vi "Launcher.vi"() -> ()   [LabVIEW 2019]
uses:
  <vilib>/ActorFramework/Message Enqueuer/Message Enqueuer.lvclass
  GUI Actor/GUI Actor.lvclass
  C:/Program Files (x86)/National Instruments/LabVIEW 2019/vi.lib/ActorFramework/Actor/Actor.lvclass
  ContadorB.lvclass
  <vilib>/ActorFramework/Message Enqueuer/Message Enqueuer.lvclass/Message Enqueuer.ctl
  <vilib>/ActorFramework/Message Enqueuer/Enqueue.vi
  <vilib>/ActorFramework/Stop Msg/Stop Msg.lvclass
  C:/Program Files (x86)/National Instruments/LabVIEW 2019/vi.lib/ActorFramework/Message/Message.lvclass
  <vilib>/ActorFramework/Message Priority Queue/Priority Enqueue.vi
  <vilib>/ActorFramework/Actor/Actor.lvclass
panel:
  in  "Actor Actual":u16(ring) items=["", "1", "2", "3", "4", "5", "6"]
  in  "Stop":bool
  in  "Actor select":enum16{"graph", "contador"}(ring)
  in  "Nuevo":bool
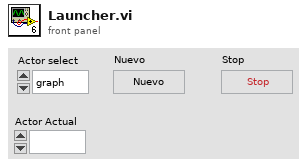
[diagram p1: front panel]
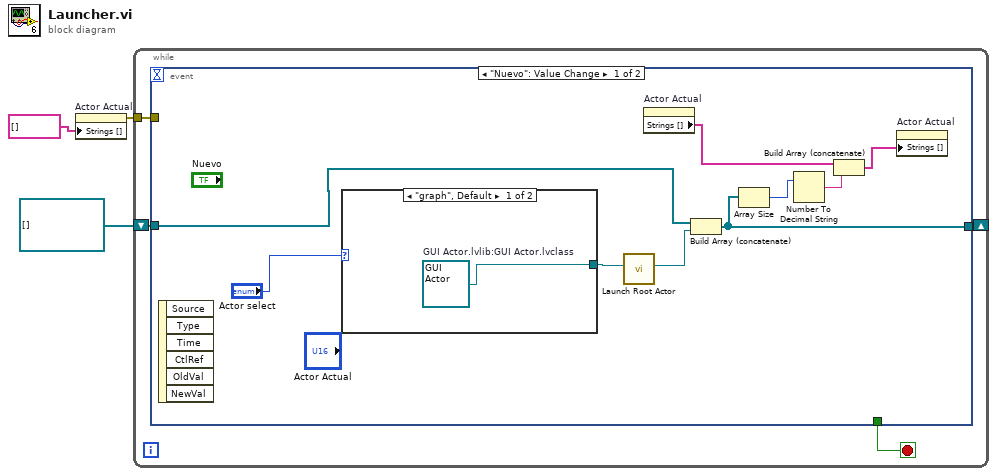
[diagram p0: block diagram]
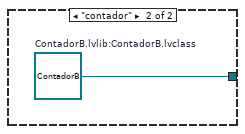
[diagram p2: hidden frame]
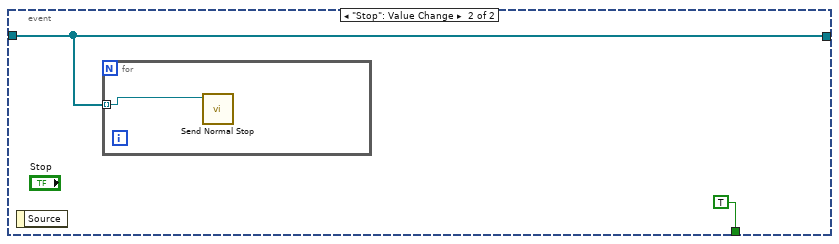
[diagram p3: hidden frame]
diagram:
  n1 = property on="Actor Actual" class="Ring (strict)"("Strings []"=string[] []) -> (error out=w1:errorcluster)  [unwired: 2 in, 1 out]
  n2 = while {
    shift-right: [w6] -> _
    shift-left: refnum<class "Message Enqueuer.lvclass">[] [] -> [w7]
    tunnel: w1 -> [w4]
    stop <- w5 stop-if-true
    n3 = event shown="[0] \"Nuevo\": Value Change" {
      selector: _ -> [_ _]
      dyn-events: _ -> [_ _]
      timeout: _ -> [_ _]
      tunnel: w7 -> [w13 w20]
      tunnel: [w12 w20] -> w6
      tunnel: [_ TRUE] -> w5
      tunnel: w4 -> [_ _]
      event "Nuevo": Value Change {
        n4 = event-data() -> ()  [unwired: 1 in, 6 out]
        n5 = case shown="\"graph\", Default" "Actor select" {
          tunnel: [w17 w18] -> w16
          frame "graph", Default {
            w17 = refnum<class "GUI Actor.lvclass"> refnum  # GUI Actor.lvlib:GUI Actor.lvclass
          }
          frame "contador" {
            w18 = refnum<class "ContadorB.lvclass"> refnum  # ContadorB.lvlib:ContadorB.lvclass
          }
        }
        n6 = call <vilib>:"Launch Root Actor.vi"("Actor"=w16) -> ("Actor's Enqueuer"=w14:refnum<class "Message Enqueuer.lvclass">)  [unwired: 9 in, 1 out]
        n7 = property on="Actor Actual" class="Ring (strict)"() -> ("Strings []"=w9:string[])  [unwired: 2 in, 2 out]
        n8 = Build Array (concatenate)(w13, w14) -> (w12:refnum<class "Message Enqueuer.lvclass">[])
        n9 = Array Size(array=w12) -> (size(s)=w11:i32)
        n10 = Number To Decimal String(number=w11) -> (decimal integer string=w10:string)  [unwired: 1 in]
        n11 = Build Array (concatenate)(w9, w10) -> (w8:string[])
        n12 = property on="Actor Actual" class="Ring (strict)"("Strings []"=w8) -> ()  [unwired: 2 in, 2 out]
      }
      event "Stop": Value Change {
        n13 = event-data() -> ()  [unwired: 1 in, 1 out]
        n14 = for {
          tunnel: w20 -> [w21] mode=indexing
          n15 = call <vilib>:"Send Normal Stop.vi"("Message Enqueuer"=w21) -> ()  [unwired: 10 in, 1 out]
        }
      }
    }
  }
